vi "lines and values.vi"(10 "DO.Lines":tag[](array[tag]), 11 "AI.PhysicalChans":tag[](array[tag])) -> (3 "Array":cluster{"Line":string, "Value":i32}[](array[cluster]))   [LabVIEW 2025, in "USB IO.lvlib" / "USB-6000.lvclass"]
uses:
  USB-6000.lvclass
  USB-6000.lvclass/USB-6000.ctl
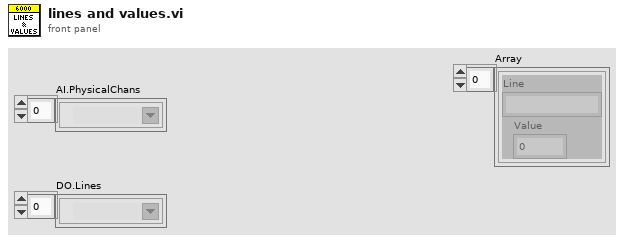
[diagram p1: front panel]
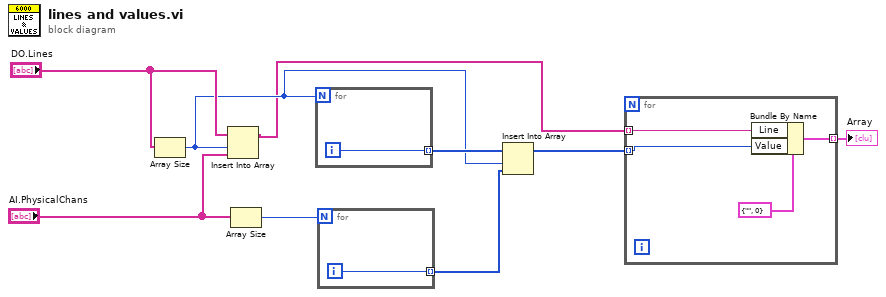
[diagram p0: block diagram]
diagram:
  n1 = Array Size(array="DO.Lines") -> (size(s)=w4:i32)
  n2 = Insert Into Array(array="DO.Lines", index=w4, new element="AI.PhysicalChans") -> (w2:tag[])
  n3 = Array Size(array="AI.PhysicalChans") -> (size(s)=w7:i32)
  n4 = for {
    N: w4 -> [_]
    tunnel: [w10] -> w6 mode=indexing
    i -> [w10]
  }
  n5 = for {
    N: w7 -> [_]
    tunnel: [w11] -> w5 mode=indexing
    i -> [w11]
  }
  n6 = Insert Into Array(array=w6, index=w4, new element=w5) -> (w3:i32[])
  n7 = for {
    tunnel: w3 -> [w12] mode=indexing
    tunnel: w2 -> [w13] mode=indexing
    tunnel: [w15] -> w1 mode=indexing
    n8 = Bundle By Name(cluster=cluster{"Line":string, "Value":i32} {"Line"="", "Value"=0}, "Line"=w13, "Value"=w12) -> (w15:cluster{"Line":string, "Value":i32})
  }
  "Array" <- w1
